vi "find timing tag indices.vi"(8 "error in":errorcluster, 10 "timing reporting":T2, 11 "data dictionary in":refnum<class "data dictionary.lvclass">) -> (0 "error out":errorcluster, 3 "reporting indices":T1={"late? index (bool)"=-1, "late count index (U32)"=-1, "dt (ns) index (U64)"=-1, "execution time (ns) index (U64)"=-1})   [LabVIEW 2013, in "Standard Engine Runtime.lvclass"]
doc: "Locates tags, if specified, for timing information. If the tags aren't found, -1 is used and that tag is disabled."
uses:
  Standard Engine Runtime.lvclass
  <vilib>/NI/Tag Bus/dictionary/data dictionary.lvclass
  Configuration/timing reporting tags.ctl
  main engine/status reporting data.ctl
  <vilib>/NI/Tag Bus/dictionary/data dictionary.lvclass/data dictionary.ctl
  <vilib>/NI/Tag Bus/dictionary/lookup polymorphs/locate Boolean.vi
  <vilib>/NI/Tag Bus/dictionary/lookup polymorphs/locate U32.vi
  <vilib>/NI/Tag Bus/dictionary/lookup polymorphs/locate U64.vi
  <vilib>/NI/Tag Bus/dictionary/search/find data index.vi
  <vilib>/NI/Tag Bus/dictionary/search/search string list.vi
  <vilib>/NI/Tag Bus/dictionary/tag not found.vi
  main engine/main engine.lvlib
  Configuration/Standard Engine Configuration.lvclass
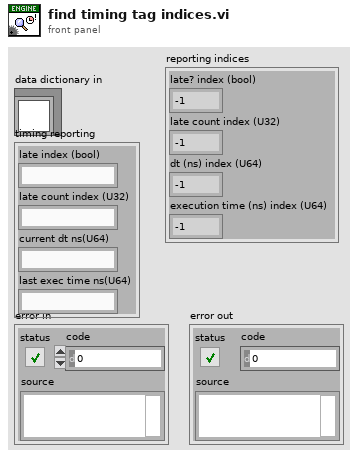
[diagram p1: front panel]
types:
  T1 = typedef "main engine.lvlib/status reporting data.ctl" = cluster{"late? index (bool)":i32, "late count index (U32)":i32, "dt (ns) index (U64)":i32, "execution time (ns) index (U64)":i32}
  T2 = typedef "Standard Engine Configuration.lvclass/timing reporting tags.ctl" = cluster{"late index (bool)":string, "late count index (U32)":string, "current dt ns(U64)":string, "last exec time ns(U64)":string}
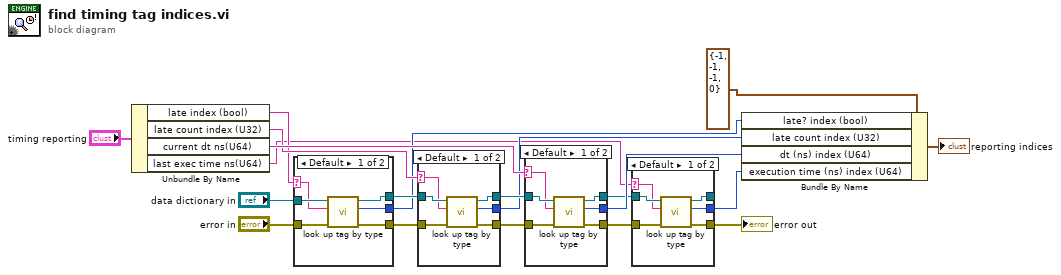
[diagram p0: block diagram]
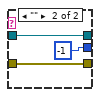
[diagram p2: hidden frame]
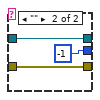
[diagram p3: hidden frame]
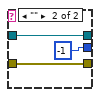
[diagram p4: hidden frame]
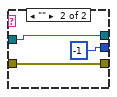
[diagram p5: hidden frame]
diagram:
  n1 = Unbundle By Name("timing reporting") -> ("late index (bool)"=w12:string, "late count index (U32)"=w18:string, "current dt ns(U64)"=w20:string, "last exec time ns(U64)"=w1:string)
  n2 = case shown="Default" w12 {
    selector: w12 -> [w22 _]
    tunnel: [w25 w29] -> w17
    tunnel: "error in" -> [w26 w29]
    tunnel: "data dictionary in" -> [w23 w28]
    tunnel: [w24 w28] -> w16
    tunnel: [w21 -1] -> w6
    frame Default {
      n3 = call-poly <vilib>:"look up tag by type.vi"("error in"=w26, "name"=w22, "data dictionary in"=w23) -> ("error out"=w25:errorcluster, "index"=w21:i32, "data dictionary out"=w24:refnum<class "data dictionary.lvclass">)  [unwired: 6 in]
    }
    frame "" {
    }
  }
  n4 = case shown="Default" w18 {
    selector: w18 -> [w31 _]
    tunnel: [w34 w38] -> w19
    tunnel: w17 -> [w35 w38]
    tunnel: w16 -> [w32 w37]
    tunnel: [w33 w37] -> w15
    tunnel: [w30 -1] -> w7
    frame Default {
      n5 = call-poly <vilib>:"look up tag by type.vi"("error in"=w35, "name"=w31, "data dictionary in"=w32) -> ("error out"=w34:errorcluster, "index"=w30:i32, "data dictionary out"=w33:refnum<class "data dictionary.lvclass">)  [unwired: 6 in]
    }
    frame "" {
    }
  }
  n6 = case shown="Default" w20 {
    selector: w20 -> [w40 _]
    tunnel: [w43 w47] -> w4
    tunnel: w19 -> [w44 w47]
    tunnel: w15 -> [w41 w46]
    tunnel: [w42 w46] -> w5
    tunnel: [w39 -1] -> w8
    frame Default {
      n7 = call-poly <vilib>:"look up tag by type.vi"("error in"=w44, "name"=w40, "data dictionary in"=w41) -> ("error out"=w43:errorcluster, "index"=w39:i32, "data dictionary out"=w42:refnum<class "data dictionary.lvclass">)  [unwired: 6 in]
    }
    frame "" {
    }
  }
  n8 = case shown="Default" w1 {
    selector: w1 -> [w49 _]
    tunnel: [w52 w56] -> w3
    tunnel: w4 -> [w53 w56]
    tunnel: w5 -> [w50 w55]
    tunnel: [w51 w55] -> _
    tunnel: [w48 -1] -> w2
    frame Default {
      n9 = call-poly <vilib>:"look up tag by type.vi"("error in"=w53, "name"=w49, "data dictionary in"=w50) -> ("error out"=w52:errorcluster, "index"=w48:i32, "data dictionary out"=w51:refnum<class "data dictionary.lvclass">)  [unwired: 6 in]
    }
    frame "" {
    }
  }
  "error out" <- w3
  n10 = Bundle By Name(cluster=T1 {"late? index (bool)"=-1, "late count index (U32)"=-1, "dt (ns) index (U64)"=-1, "execution time (ns) index (U64)"=0} ("status reporting"), "late? index (bool)"=w6, "late count index (U32)"=w7, "dt (ns) index (U64)"=w8, "execution time (ns) index (U64)"=w2) -> (→"reporting indices":T1)
